vi "Wind Turbine Get Turbine Speed.vi"(0 "Data Refnum":T1, 11 "error in (no error)":errorcluster) -> (4 "Data Refnum out":T1, 6 "Turbine Speed (RPM)":dbl, 15 "error out":errorcluster)   [LabVIEW 2011, in "SEQ - Solution.lvlib"]
doc: "One VI in the solution for the Wind Turbine class. This group of VIs is built on the SEQ design pattern and illustrates the power of references and named queues.\n\nAAL 9/09"
uses:
  SEQ - Solution.lvlib
  Controls/Wind Turbine DataRef.ctl
  Controls/Wind Turbine Data.ctl
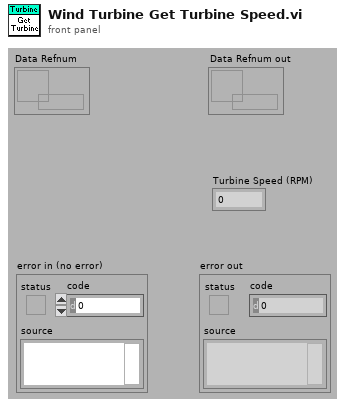
[diagram p1: front panel]
types:
  T1 = typedef "SEQ - Solution.lvlib/Wind Turbine DataRef.ctl" = refnum<queue>
  T2 = typedef "SEQ - Solution.lvlib/Wind Turbine Data.ctl" = cluster{" Wind Speed (ms)":dbl, "Turbine Speed (RPM)":dbl, "Angle Attack (Degs.)":dbl, "Current Power (kW)":dbl, "Energy Generation (kW*hr)":dbl}
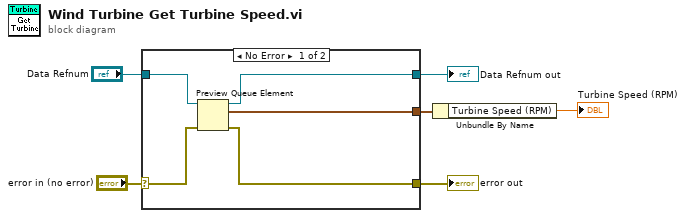
[diagram p0: block diagram]
diagram:
  n1 = case shown="No Error" "error in (no error)" {
    selector: "error in (no error)" -> [w10 w13]
    tunnel: [w8 w13] -> w5
    tunnel: "Data Refnum" -> [w11 w12]
    tunnel: [w9 w12] -> w4
    tunnel: [w7 _] -> w2
    frame No Error {
      n2 = Preview Queue Element(queue=w11, error in (no error)=w10) -> (queue out=w9:T1, element=w7:T2, error out=w8:errorcluster)  [unwired: 1 in, 1 out]
    }
    frame Error {
    }
  }
  "error out" <- w5
  "Data Refnum out" <- w4
  n3 = Unbundle By Name(w2) -> ("Turbine Speed (RPM)"=→"Turbine Speed (RPM)":dbl)
